vi "Draw BER Curve.vi"(6 "Sample Step":dbl=1.0, 7 "Samples":i32=30, 9 "Message Bits":i32=500) -> ()   [LabVIEW 2013]
panel:
  out "Curves":dbl[][](graph)
  in  "Averaging Number":i32=100
  in  "Initial Value":i32
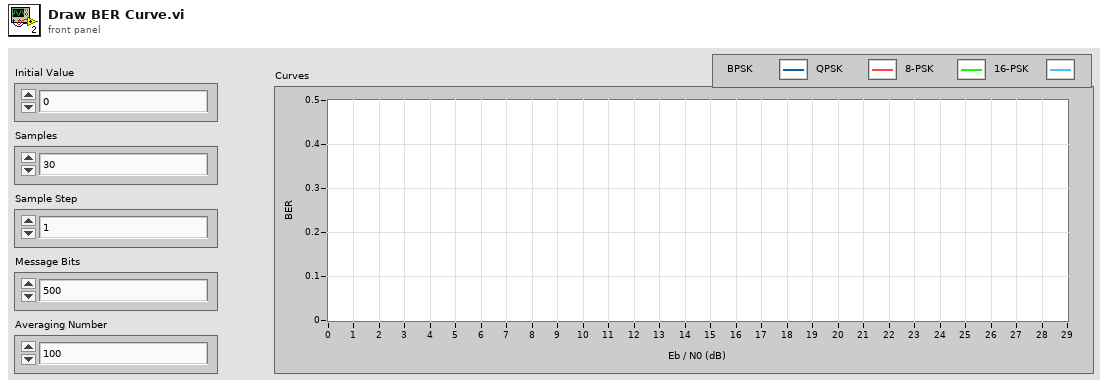
[diagram p1: front panel]
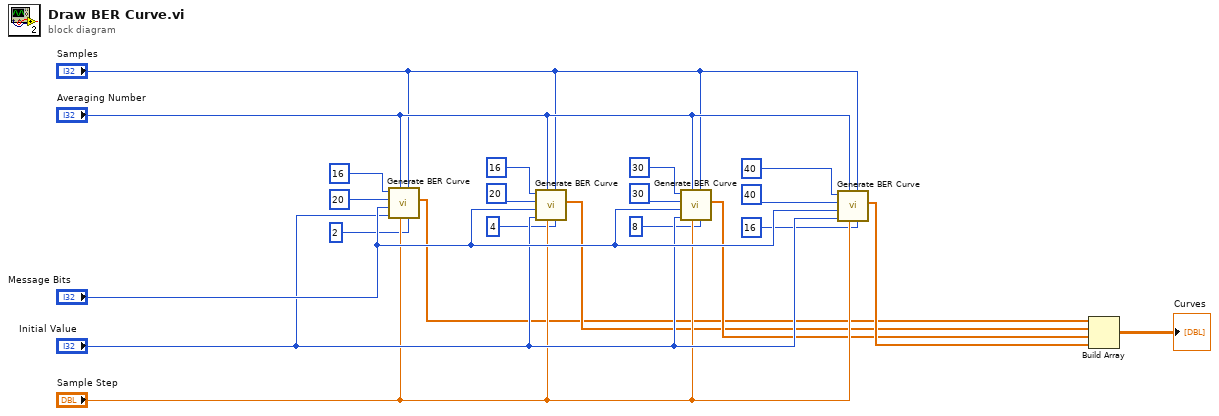
[diagram p0: block diagram]
diagram:
  n1 = call "Generate BER Curve.vi"("M-PSK"=2, "Samples"="Samples", "Sample Step"="Sample Step", "Averaging Number"="Averaging Number", "Initial Value"="Initial Value", "Message Bits"="Message Bits", "Synchronization Sequence"=20, "Zero Pad"=16) -> ("BER Curve"=w15:dbl[])  [unwired: 3 out]
  n2 = call "Generate BER Curve.vi"("M-PSK"=4, "Samples"="Samples", "Sample Step"="Sample Step", "Averaging Number"="Averaging Number", "Initial Value"="Initial Value", "Message Bits"="Message Bits", "Synchronization Sequence"=20, "Zero Pad"=16) -> ("BER Curve"=w16:dbl[])  [unwired: 3 out]
  n3 = call "Generate BER Curve.vi"("M-PSK"=8, "Samples"="Samples", "Sample Step"="Sample Step", "Averaging Number"="Averaging Number", "Initial Value"="Initial Value", "Message Bits"="Message Bits", "Synchronization Sequence"=30, "Zero Pad"=30) -> ("BER Curve"=w17:dbl[])  [unwired: 3 out]
  n4 = call "Generate BER Curve.vi"("M-PSK"=16, "Samples"="Samples", "Sample Step"="Sample Step", "Averaging Number"="Averaging Number", "Initial Value"="Initial Value", "Message Bits"="Message Bits", "Synchronization Sequence"=40, "Zero Pad"=40) -> ("BER Curve"=w18:dbl[])  [unwired: 3 out]
  n5 = Build Array(w15, w16, w17, w18) -> (→"Curves":dbl[][])
